vi "Recurse Through Project Items.vi"(6 "FPGA":string, 7 "FPGA Resource":string, 8 "error in (no error)":errorcluster, 9 "IO in":variant, 10 "Modules in":variant, 11 "ProjectItem in":refnum<vi>) -> (0 "error out":errorcluster, 1 "IO out":variant, 2 "Modules out":variant)   [LabVIEW 2025, in "Project.lvclass"]
uses:
  Project.lvclass
  Elemental IO Properties.ctl
  <vilib>/Utility/error.llb/Trim Whitespace One-Sided.vi
  Project.lvclass/Project.ctl
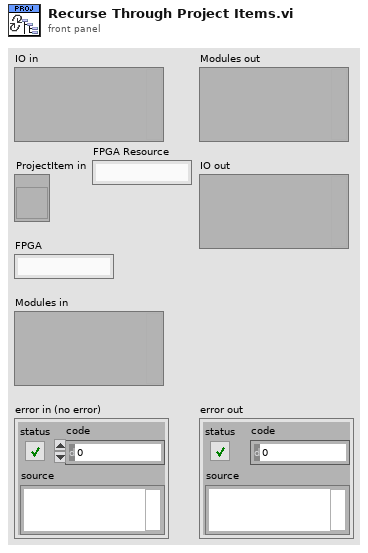
[diagram p1: front panel]
types:
  T1 = typedef "Project.lvclass/Elemental IO Properties.ctl" = cluster{"FPGA Name":string, "Group":string, "IO Resource":string, "IO Name":string, "FPGA Resource":string}
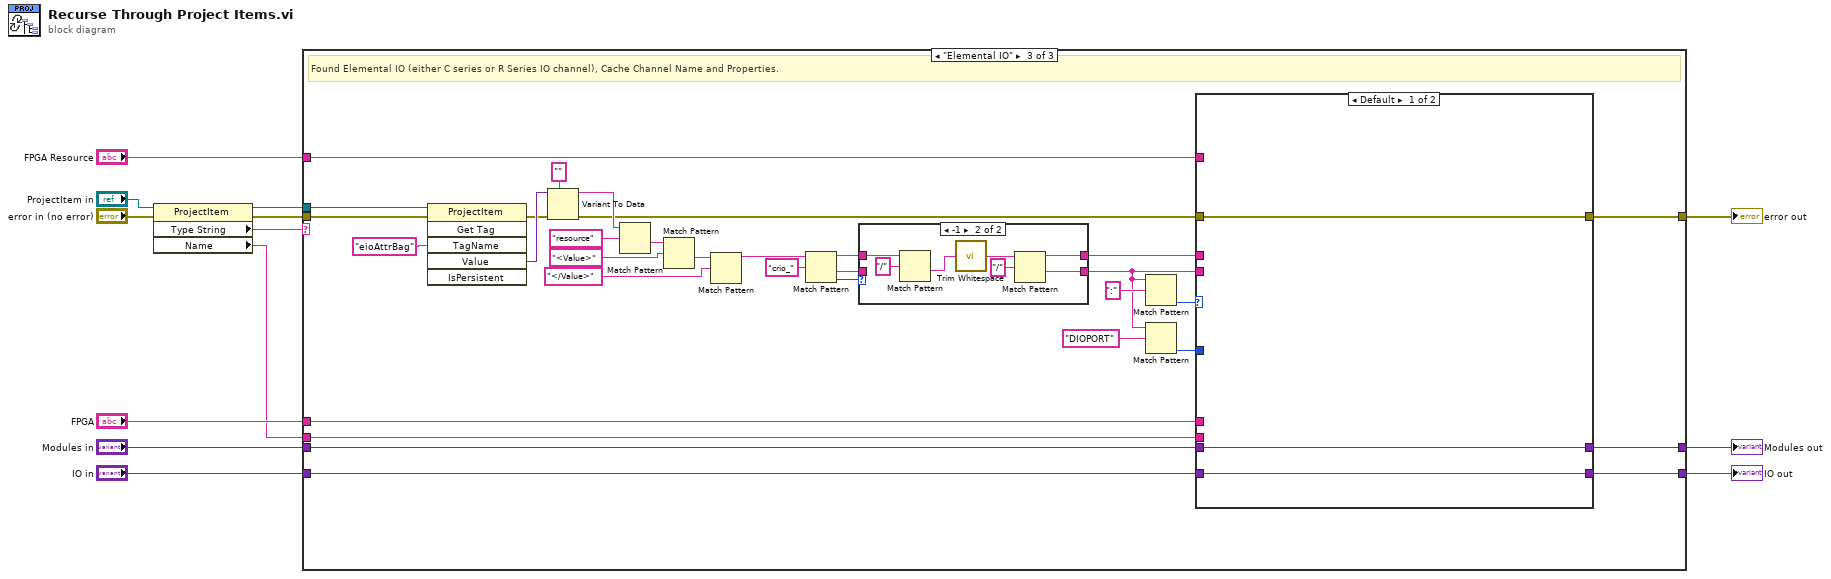
[diagram p0: block diagram]
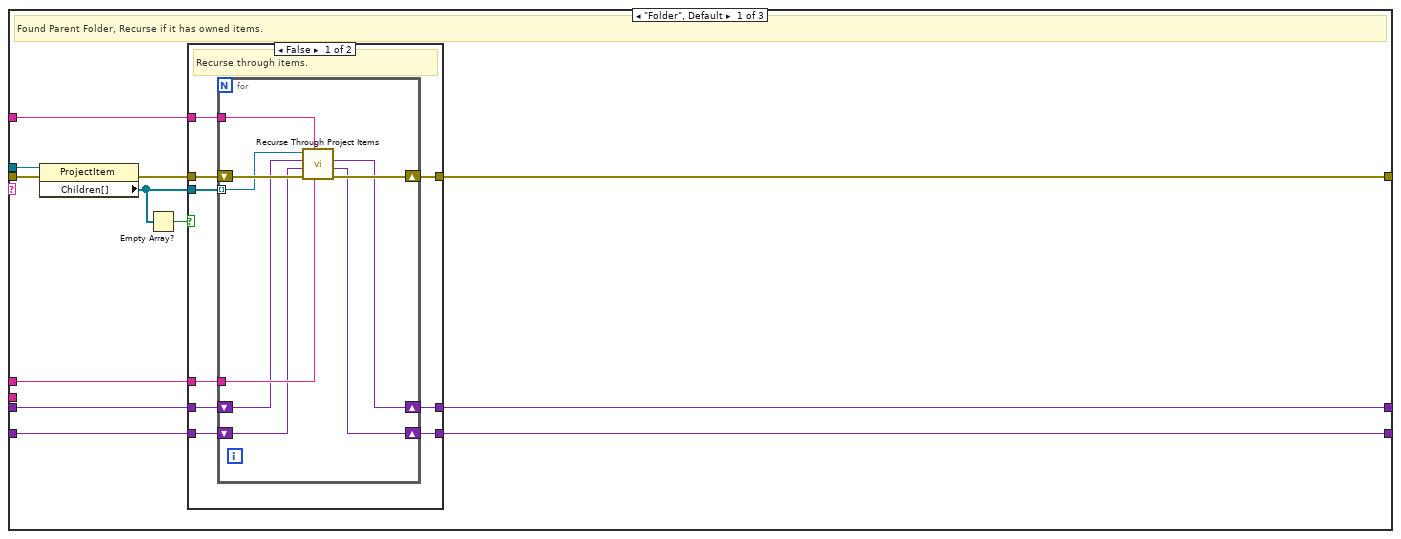
[diagram p2: hidden frame]
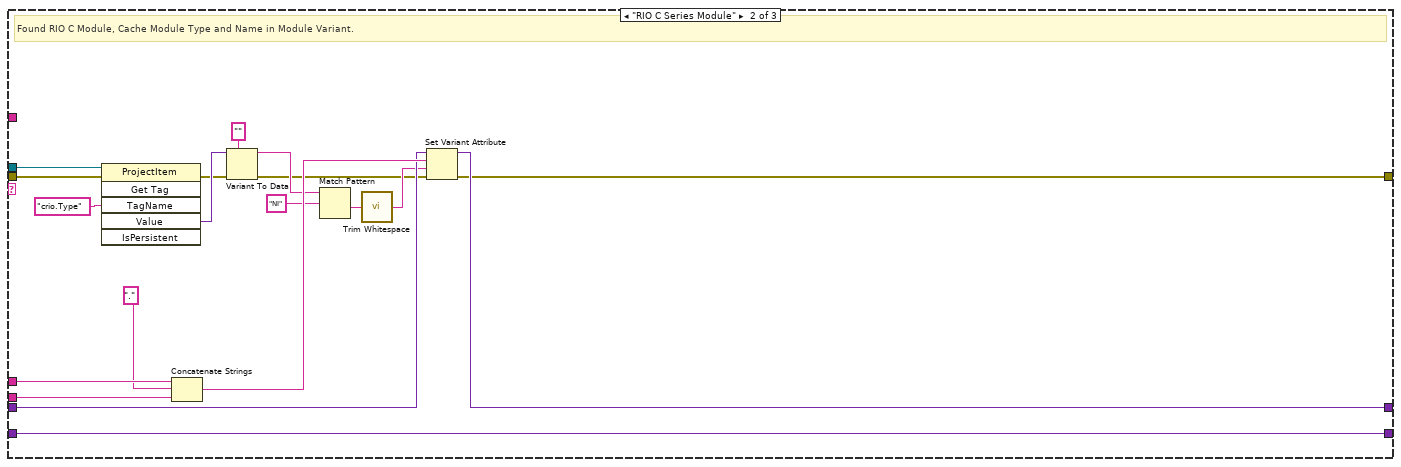
[diagram p4: hidden frame]
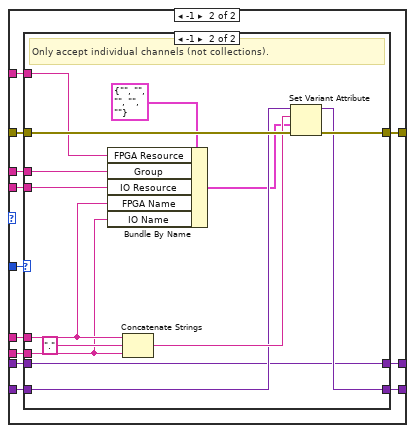
[diagram p5: hidden frame]
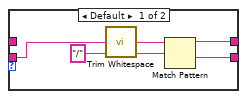
[diagram p7: hidden frame]
diagram:
  n1 = property class="ProjectItem"(reference="ProjectItem in", error in="error in (no error)") -> (reference out=w5:refnum<vi>, error out=w6:errorcluster, "Type String"=w4:string, "Name"=w8:string)
  n2 = case shown="\"Elemental IO\"" w4 {
    tunnel: w5 -> [w25 w65 w97]
    tunnel: w6 -> [w24 w63 w96]
    tunnel: [w20 w48 w84] -> w7
    tunnel: w8 -> [_ w57 w79]
    tunnel: "FPGA" -> [w19 w59 w80]
    tunnel: "Modules in" -> [w18 w55 w69]
    tunnel: [w15 w54 w70] -> w11
    tunnel: "IO in" -> [w17 w47 w83]
    tunnel: [w16 w47 w82] -> w13
    tunnel: "FPGA Resource" -> [w14 _ w73]
    frame "Folder", Default {
      # "Found Parent Folder, Recurse if it has owned items."
      n3 = property class="ProjectItem"(reference=w25, error in=w24) -> (error out=w22:errorcluster, "Children[]"=w21:refnum<vi>[])  [unwired: 1 out]
      n4 = Empty Array?(array=w21) -> (empty?=w23:bool)
      n5 = case shown="False" w23 {
        tunnel: w22 -> [w34 w46]
        tunnel: w21 -> [w33 _]
        tunnel: [w32 w46] -> w20
        tunnel: w19 -> [w31 _]
        tunnel: w18 -> [w30 w44]
        tunnel: w17 -> [w29 w45]
        tunnel: [w28 w45] -> w16
        tunnel: [w27 w44] -> w15
        tunnel: w14 -> [w26 _]
        frame False {
          # "Recurse through items."
          n6 = for {
            tunnel: w33 -> [w42] mode=indexing
            shift-right: [w40] -> w32
            shift-left: w34 -> [w43]
            tunnel: w31 -> [w41]
            shift-right: [w36] -> w27
            shift-left: w30 -> [w39]
            shift-right: [w37] -> w28
            shift-left: w29 -> [w38]
            tunnel: w26 -> [w35]
            n7 = call "Recurse Through Project Items.vi"("FPGA"=w41, "FPGA Resource"=w35, "error in (no error)"=w43, "IO in"=w38, "Modules in"=w39, "ProjectItem in"=w42) -> ("error out"=w40:errorcluster, "IO out"=w37:variant, "Modules out"=w36:variant)  [unwired: 3 in]
          }
        }
        frame True {
          # "No items, do nothing."
        }
      }
    }
    frame "RIO C Series Module" {
      # "Found RIO C Module, Cache Module Type and Name in Module Variant."
      n8 = invoke class="ProjectItem" method="Get Tag"(reference=w65, error in=w63, "TagName"="crio.Type" ("Tag Name")) -> (error out=w61:errorcluster, "Value"=w62:variant)  [unwired: 3 in, 4 out]
      n9 = Concatenate Strings(w59, "." ("string"), w57) -> (w56:string)
      n10 = Variant To Data(error in=w61, type="", Variant=w62) -> (data=w53:string, error out=w49:errorcluster)
      n11 = Match Pattern(string=w53, regular expression="NI") -> (after substring=w52:string)  [unwired: 1 in, 3 out]
      n12 = call <vilib>:"Trim Whitespace.vi"("string"=w52) -> ("trimmed string"=w50:string)  [unwired: 1 in]
      n13 = Set Variant Attribute(Variant=w55, name=w56, value=w50, error in=w49) -> (Variant out=w54:variant, error out=w48:errorcluster)  [unwired: 1 out]
    }
    frame "Elemental IO" {
      # "Found Elemental IO (either C series or R Series IO channel), Cache Channel Name and Properties."
      n14 = invoke class="ProjectItem" method="Get Tag"(reference=w97, error in=w96, "TagName"="eioAttrBag" ("Tag Name")) -> (error out=w91:errorcluster, "Value"=w94:variant)  [unwired: 3 in, 4 out]
      n15 = Variant To Data(error in=w91, type="" ("Tag Name"), Variant=w94) -> (data=w92:string, error out=w85:errorcluster)
      n16 = Match Pattern(string=w92, regular expression="resource") -> (after substring=w89:string)  [unwired: 1 in, 3 out]
      n17 = Match Pattern(string=w89, regular expression="<Value>") -> (after substring=w87:string)  [unwired: 1 in, 3 out]
      n18 = Match Pattern(string=w87, regular expression="</Value>") -> (before substring=w78:string)  [unwired: 1 in, 3 out]
      n19 = Match Pattern(string=w78, regular expression="crio_") -> (before substring=w74:string, after substring=w75:string, offset past match=w76:i32)  [unwired: 1 in, 1 out]
      n20 = case shown="-1" w76 {
        tunnel: [w132 w139] -> w81
        tunnel: [w131 w138] -> w68
        tunnel: w75 -> [w130 _]
        tunnel: w74 -> [_ w135]
        frame Default {
          n21 = call <vilib>:"Trim Whitespace.vi"("string"=w130) -> ("trimmed string"=w134:string)  [unwired: 1 in]
          n22 = Match Pattern(string=w134, regular expression="/") -> (before substring=w132:string, after substring=w131:string)  [unwired: 1 in, 2 out]
        }
        frame -1 {
          n23 = Match Pattern(string=w135, regular expression="/") -> (after substring=w136:string)  [unwired: 1 in, 3 out]
          n24 = call <vilib>:"Trim Whitespace.vi"("string"=w136) -> ("trimmed string"=w141:string)  [unwired: 1 in]
          n25 = Match Pattern(string=w141, regular expression="/") -> (before substring=w139:string, after substring=w138:string)  [unwired: 1 in, 2 out]
        }
      }
      n26 = Match Pattern(string=w68, regular expression=":") -> (offset past match=w71:i32)  [unwired: 1 in, 3 out]
      n27 = Match Pattern(string=w68, regular expression="DIOPORT") -> (offset past match=w66:i32)  [unwired: 1 in, 3 out]
      n28 = case shown="Default" w71 {
        tunnel: w85 -> [w100 w112]
        tunnel: [w100 w111] -> w84
        tunnel: w83 -> [w99 w110]
        tunnel: [w99 w109] -> w82
        tunnel: w81 -> [_ w108]
        tunnel: w80 -> [_ w107]
        tunnel: w79 -> [_ w106]
        tunnel: w73 -> [_ w105]
        tunnel: w68 -> [_ w104]
        tunnel: [w98 w102] -> w70
        tunnel: w69 -> [w98 w101]
        tunnel: w66 -> [_ w103]
        frame Default {
        }
        frame -1 {
          n29 = case shown="-1" w103 {
            tunnel: w112 -> [w113 w129]
            tunnel: [w113 w128] -> w111
            tunnel: w110 -> [w115 w126]
            tunnel: [w115 w125] -> w109
            tunnel: w108 -> [_ w122]
            tunnel: w107 -> [_ w121]
            tunnel: w106 -> [_ w119]
            tunnel: w105 -> [_ w118]
            tunnel: w104 -> [_ w117]
            tunnel: [w114 w116] -> w102
            tunnel: w101 -> [w114 w116]
            frame Default {
            }
            frame -1 {
              # "Only accept individual channels (not collections)."
              n30 = Bundle By Name(cluster=T1 {"FPGA Name"="", "Group"="", "IO Resource"="", "IO Name"="", "FPGA Resource"=""}, "FPGA Resource"=w118, "Group"=w122, "IO Resource"=w117, "FPGA Name"=w121, "IO Name"=w119) -> (w120:T1)
              n31 = Concatenate Strings(w121, "." ("string"), w119) -> (w127:string)
              n32 = Set Variant Attribute(Variant=w126, name=w127, value=w120, error in=w129) -> (Variant out=w125:variant, error out=w128:errorcluster)  [unwired: 1 out]
            }
          }
        }
      }
    }
  }
  "IO out" <- w13
  "Modules out" <- w11
  "error out" <- w7
